vi "AB_Version_Path.vi"(10 "buildVersion":T1, 11 "unversioned path":path) -> (3 "versioned path":path)   [LabVIEW 2020]
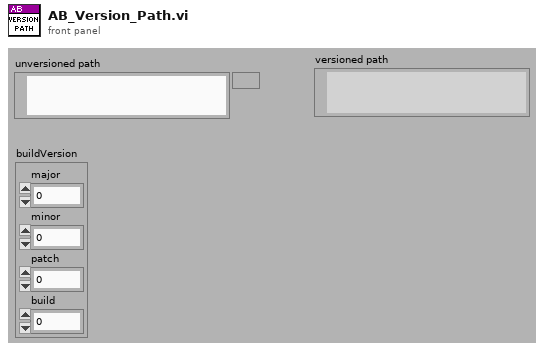
[diagram p1: front panel]
types:
  T1 = cluster{"major":u16, "minor":u16, "patch":u16, "build":u16}
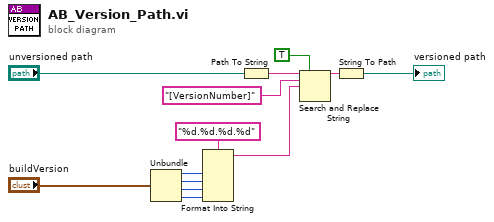
[diagram p0: block diagram]
diagram:
  n1 = Unbundle("buildVersion") -> ("major"=w8:u16, "minor"=w7:u16, "patch"=w6:u16, "build"=w5:u16)
  n2 = Format Into String(format string="%d.%d.%d.%d", w8, w7, w6, w5) -> (resulting string=w4:string)  [unwired: 2 in, 1 out]
  n3 = Path To String(path="unversioned path") -> (string=w11:string)
  n4 = Search and Replace String(replace all?=TRUE ("replace all? (F)"), input string=w11, search string="[VersionNumber]", replace string=w4) -> (result string=w13:string)  [unwired: 4 in, 3 out]
  n5 = String To Path(string=w13) -> (path=→"versioned path":path)
